vi "oax_Generate Amplitude Modulated Signal (block).vi"(5 "reset?":bool, 7 "fs":dbl, 8 "phase in":dbl, 9 "envelop config":T1={"f"=0.4, "high limit"=8.0, "low limit"=1.0} {"low limit" format="%.2f"; "high limit" format="%.2f"; "f" format="%.2f"}, 10 "AM selection":u16(ring) items=["None", "Sine", "Triangle"], 11 "x":dbl[](array[numeric])) -> (0 "phase out":dbl format="%0.2e", 3 "AM modulated signal":dbl[](array[numeric]))   [LabVIEW 2017]
uses:
  <vilib>/Analysis/NI_AALBase.lvlib
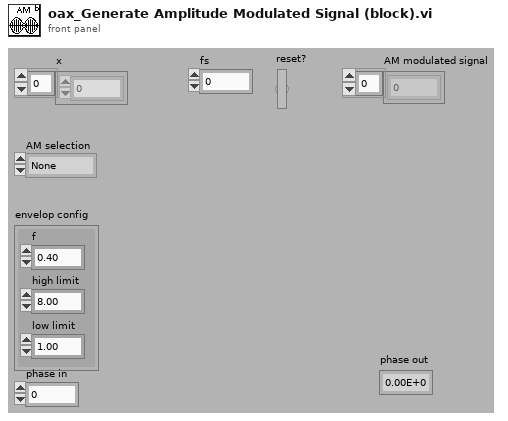
[diagram p1: front panel]
types:
  T1 = cluster{"f":dbl, "high limit":dbl, "low limit":dbl}
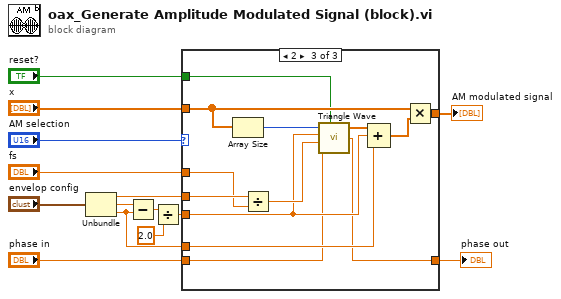
[diagram p0: block diagram]
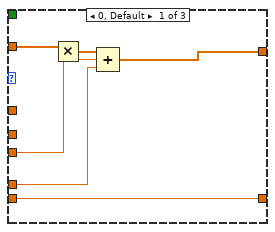
[diagram p2: hidden frame]
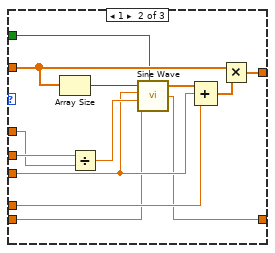
[diagram p3: hidden frame]
diagram:
  n1 = Unbundle("envelop config") -> ("f"=w5:dbl, "high limit"=w11:dbl, "low limit"=w7:dbl)
  n2 = Subtract(x=w11, y=w7) -> (x-y=w10:dbl)
  n3 = Divide(x=w10, y=2.0) -> (x/y=w8:dbl)
  n4 = case shown="2" "AM selection" {
    tunnel: "x" -> [w20 w27 w40]
    tunnel: w8 -> [w16 w24 w37]
    tunnel: w7 -> [w17 w28 w41]
    tunnel: [w18 w25 w38] -> w6
    tunnel: w5 -> [_ w32 w45]
    tunnel: "fs" -> [_ w31 w44]
    tunnel: "reset?" -> [_ w23 w36]
    tunnel: "phase in" -> [w15 w22 w35]
    tunnel: [w15 w21 w34] -> w1
    frame 0, Default {
      n5 = Multiply(x=w20, y=w16) -> (x*y=w19:dbl[])
      n6 = Compound Arithmetic op=ADD(w19, w16, w17) -> (w18:dbl[])
    }
    frame 1 {
      n7 = Array Size(array=w27) -> (size(s)=w33:i32)
      n8 = Divide(x=w32, y=w31) -> (x/y=w29:dbl)
      n9 = call <vilib>:"Sine Wave.vi"("samples"=w33, "amplitude"=w24, "frequency"=w29, "phase in"=w22, "reset phase"=w23) -> ("sine wave"=w30:dbl[], "phase out"=w21:dbl)  [unwired: 1 out]
      n10 = Compound Arithmetic op=ADD(w30, w24, w28) -> (w26:dbl[])
      n11 = Multiply(x=w27, y=w26) -> (x*y=w25:dbl[])
    }
    frame 2 {
      n12 = Array Size(array=w40) -> (size(s)=w46:i32)
      n13 = Divide(x=w45, y=w44) -> (x/y=w42:dbl)
      n14 = call <vilib>:"Triangle Wave.vi"("samples"=w46, "amplitude"=w37, "frequency"=w42, "phase in"=w35, "reset phase"=w36) -> ("triangle wave"=w43:dbl[], "phase out"=w34:dbl)  [unwired: 1 out]
      n15 = Compound Arithmetic op=ADD(w43, w37, w41) -> (w39:dbl[])
      n16 = Multiply(x=w40, y=w39) -> (x*y=w38:dbl[])
    }
  }
  "AM modulated signal" <- w6
  "phase out" <- w1
